vi "Initialize.vi"(8 "error in (no error)":errorcluster, 11 "MQTT-Server in":refnum<class "MQTT-Server.lvclass">) -> (0 "error out":errorcluster, 1 "MQTT_Base out":refnum<class "Server.lvclass">, 2 "Event Ref":refnum<event-registration>, 3 "MQTT-Server out":refnum<class "MQTT-Server.lvclass">)   [LabVIEW 2023, in "MQTT-Server.lvlib" / "MQTT-Server.lvclass"]
uses:
  MQTT-Server.lvclass
  <vilib>/G Open Source Project for LabVIEW/MQTT Broker/Server class/Server.lvclass
  C:/Program Files/National Instruments/LabVIEW 2023/vi.lib/LabVIEW Open Source Project/MQTT Connection/MQTT_Base/Base Class/MQTT_Base.lvclass
  <vilib>/G Open Source Project for LabVIEW/MQTT Broker/Server class/Public Events -- cluster.ctl
  <vilib>/G Open Source Project for LabVIEW/MQTT Broker/ConnectionHandler/Client Event -- cluster.ctl
  <vilib>/G Open Source Project for LabVIEW/MQTT Broker/ConnectionHandler/Client Action -- enum.ctl
  <vilib>/LabVIEW Open Source Project/MQTT Control Packets/Control Packets/PUBLISH/PUBLISH.lvclass
  CustomFlat/CustomFlat.lvclass
  C:/Program Files/National Instruments/LabVIEW 2023/vi.lib/LabVIEW Open Source Project/OpenSerializer/Serializer/Serializer.lvclass
  MQTT-Server.lvclass/MQTT-Server.ctl
  <vilib>/LabVIEW Open Source Project/MQTT Connection/MQTT_Base/Base Class/MQTT_Base.lvclass/MQTT_Base.ctl
  <vilib>/G Open Source Project for LabVIEW/MQTT Broker/Server class/Server.lvclass/Server.ctl
  <vilib>/LabVIEW Open Source Project/Connection/Connection.TCP/Connection.TCP.lvclass
  C:/Program Files/National Instruments/LabVIEW 2023/vi.lib/LabVIEW Open Source Project/Connection/Connection/Connection.lvclass
  <vilib>/LabVIEW Open Source Project/OpenSerializer/Serializer.FlattenedString/Serializer.FlattenedString.lvclass
  <vilib>/LabVIEW Open Source Project/OpenSerializer/Serializer/Serializer.lvclass
  <vilib>/LabVIEW Open Source Project/MQTT Connection/MQTT_Base/Base Class/MQTT_Base.lvclass
  C:/Program Files/National Instruments/LabVIEW 2023/vi.lib/G Open Source Project for LabVIEW/MQTT Broker/Server class/Server.lvclass
  C:/Program Files/National Instruments/LabVIEW 2023/vi.lib/LabVIEW Open Source Project/Connection/Connection.TCP/Connection.TCP.lvclass
  C:/Users/KIV4BP/Documents/Projects/mqtt-budlug/source/CustomFlat/CustomFlat.lvclass
  <vilib>/G Open Source Project for LabVIEW/MQTT Broker/ConnectionHandler/ConnectionHandler.lvclass
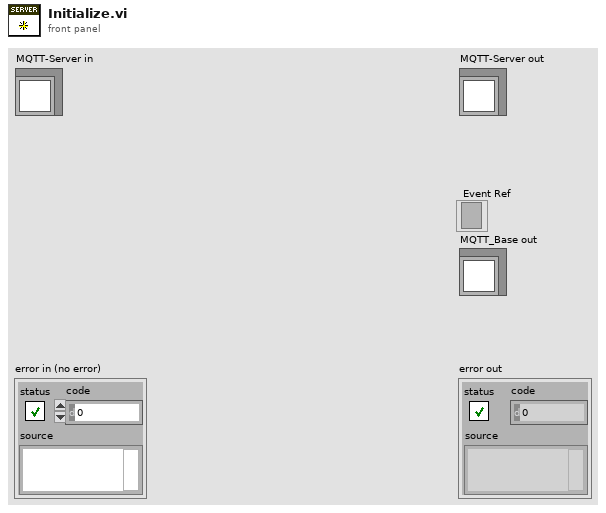
[diagram p1: front panel]
types:
  T1 = typedef "MQTT Base.lvlib/MQTT_Base.lvclass/Public Events -- cluster.ctl" = cluster{"Stop Event":refnum<user-event>, "Error Event":refnum<user-event>, "Inbound Message":refnum<user-event>}
  T2 = typedef "MQTT Server.lvlib/Server.lvclass/Public Events -- cluster.ctl" = cluster{"NbConnections":refnum<user-event>, "Client Event":refnum<user-event>}
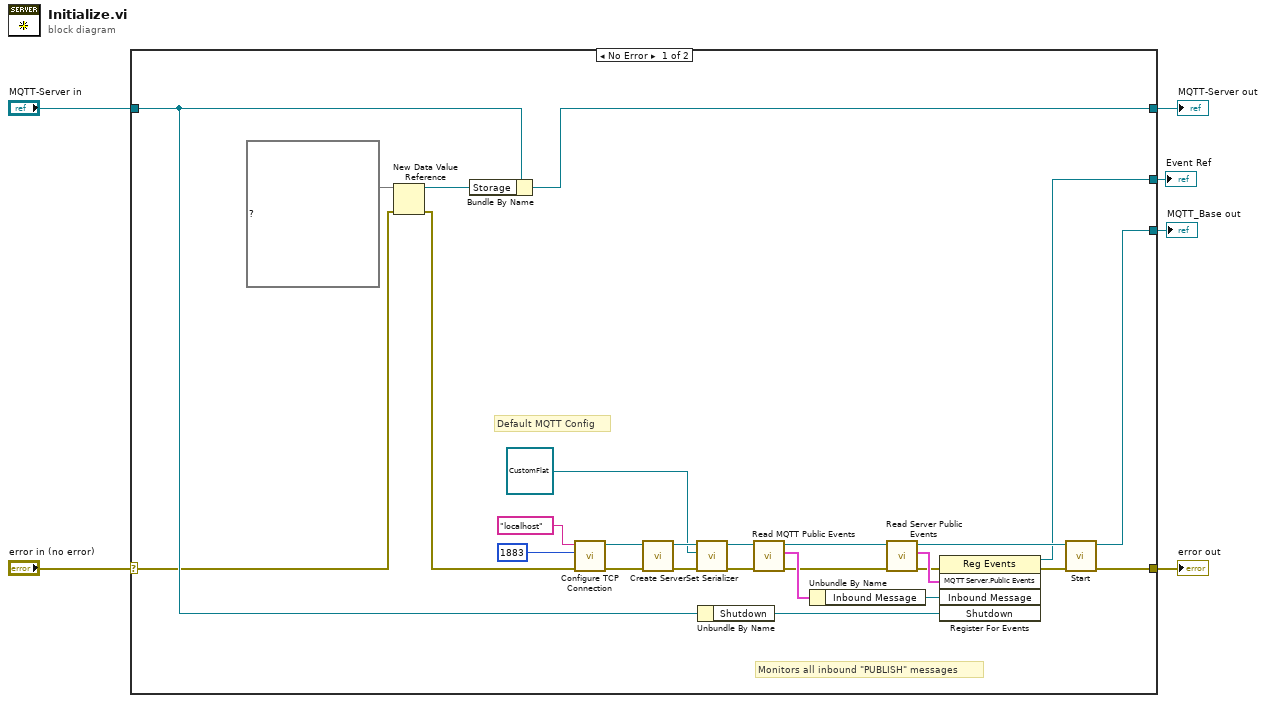
[diagram p0: block diagram]
diagram:
  n1 = case shown="No Error" "error in (no error)" {
    selector: "error in (no error)" -> [w9 w35]
    tunnel: [w15 w35] -> w5
    tunnel: [w8 w34] -> w3
    tunnel: "MQTT-Server in" -> [w10 w34]
    tunnel: [w14 _] -> w2
    tunnel: [w13 _] -> w1
    frame No Error {
      # "Default MQTT Config"
      # "Monitors all inbound \"PUBLISH\" messages"
      n2 = New Data Value Reference(data value=map{string, waveform(dbl)} {} ("Storage"), error in=w9) -> (data value reference=w11:refnum<data-value>, error out=w7:errorcluster)
      n3 = Bundle By Name(cluster=w10, "Storage"=w11) -> (w8:refnum<class "MQTT-Server.lvclass">)
      n4 = call <vilib>:"Configure TCP Connection.vi"("error in (no error)"=w7, "remote port (80)"=u16 1883, "address (localhost)"="localhost") -> ("error out"=w22:errorcluster, "Connection.TCP"=w33:refnum<class "Connection.TCP.lvclass">)  [unwired: 7 in]
      n5 = call <vilib>:"Create Server.vi"("error in (no error)"=w22, "Connection Configuration"=w33) -> ("error out"=w20:errorcluster, "Server"=w19:refnum<class "Server.lvclass">)  [unwired: 8 in]
      n6 = call <vilib>:"Set Serializer.vi"("error in (no error)"=w20, "Serializer (default: Flattened String)"=refnum<class "CustomFlat.lvclass"> refnum ("CustomFlat.lvclass"), "MQTT_Base"=w19) -> ("error out"=w17:errorcluster, "MQTT_Base out"=w18:refnum<class "Server.lvclass">)  [unwired: 7 in]
      n7 = Unbundle By Name(w10) -> ("Shutdown"=w21:refnum<user-event>)
      n8 = call <vilib>:"Read MQTT Public Events.vi"("error in (no error)"=w17, "MQTT_Base in"=w18) -> ("error out"=w30:errorcluster, "MQTT Public Events"=w31:T1, "MQTT_Base out"=w29:refnum<class "Server.lvclass">)  [unwired: 7 in]
      n9 = Unbundle By Name(w31) -> ("Inbound Message"=w32:refnum<user-event>)
      n10 = call <vilib>:"Read Server Public Events.vi"("error in (no error)"=w30, "Server in"=w29) -> ("error out"=w25:errorcluster, "MQTT Server.Public Events"=w26:T2, "Server out"=w27:refnum<class "Server.lvclass">)  [unwired: 7 in]
      n11 = register-events(error in=w25, w26, w32, w21) -> (reference out=w13:refnum<event-registration>, error out=w28:errorcluster)  [unwired: 1 in]
      n12 = call <vilib>:"Start.vi"("error in (no error)"=w28, "MQTT_Base in"=w27) -> ("error out"=w15:errorcluster, "MQTT_Base out"=w14:refnum<class "Server.lvclass">)  [unwired: 7 in, 1 out]
    }
    frame Error {
    }
  }
  "error out" <- w5
  "MQTT-Server out" <- w3
  "MQTT_Base out" <- w2
  "Event Ref" <- w1
